vi "Untitled 7.vi"() -> ()   [LabVIEW 2019]
uses:
  <vilib>/Utility/file.llb/Read Delimited Spreadsheet (string).vi
panel:
  out "subarray 2":dbl[](array[numeric])=[0.124575, 0.249206, 0.374163, 0.498874, 0.623563, 0.748281, 0.872983, 0.997694, 1.12241, 1.247065, 1.371768, 1.496488, 1.621191, 1.745701, 1.870395, 1.995091, 2.119804, 2.244506, 2.369205]
  out "subarray":dbl[](array[numeric])=[204.971, 409.1489, 614.1025, 818.3818, 1022.829, 1226.951, 1431.292, 1635.939, 1840.247, 2044.703, 2248.928, 2453.218, 2657.61, 2861.815, 3066.024, 3270.177, 3474.445, 3679.15, 3883.288]
  out "appended array":string[][](array[string])=[["204.9710", "0.124575"], ["409.1489", "0.249206"], ["614.1025", "0.374163"], ["818.3818", "0.498874"], ["1022.829", "0.623563"], ["1226.951", "0.748281"], ["1431.292", "0.872983"], ["1635.939", "0.997694"], ["1840.247", "1.122410"], ["2044.703", "1.247065"], ["2248.928", "1.371768"], ["2453.218", "1.496488"], ["2657.610", "1.621191"], ["2861.815", "1.745701"], ["3066.024", "1.870395"], ["3270.177", "1.995091"], ["3474.445", "2.119804"], ["3679.150", "2.244506"], ["3883.288", "2.369205"]]
  out "all rows":string[][](array[string])
  in  "file path (dialog if empty)":path=path "D:/Projects/C2000/Grande/Data/ADC/Offset_Gain/Int_Ref_FCS_CHIP-2.txt"
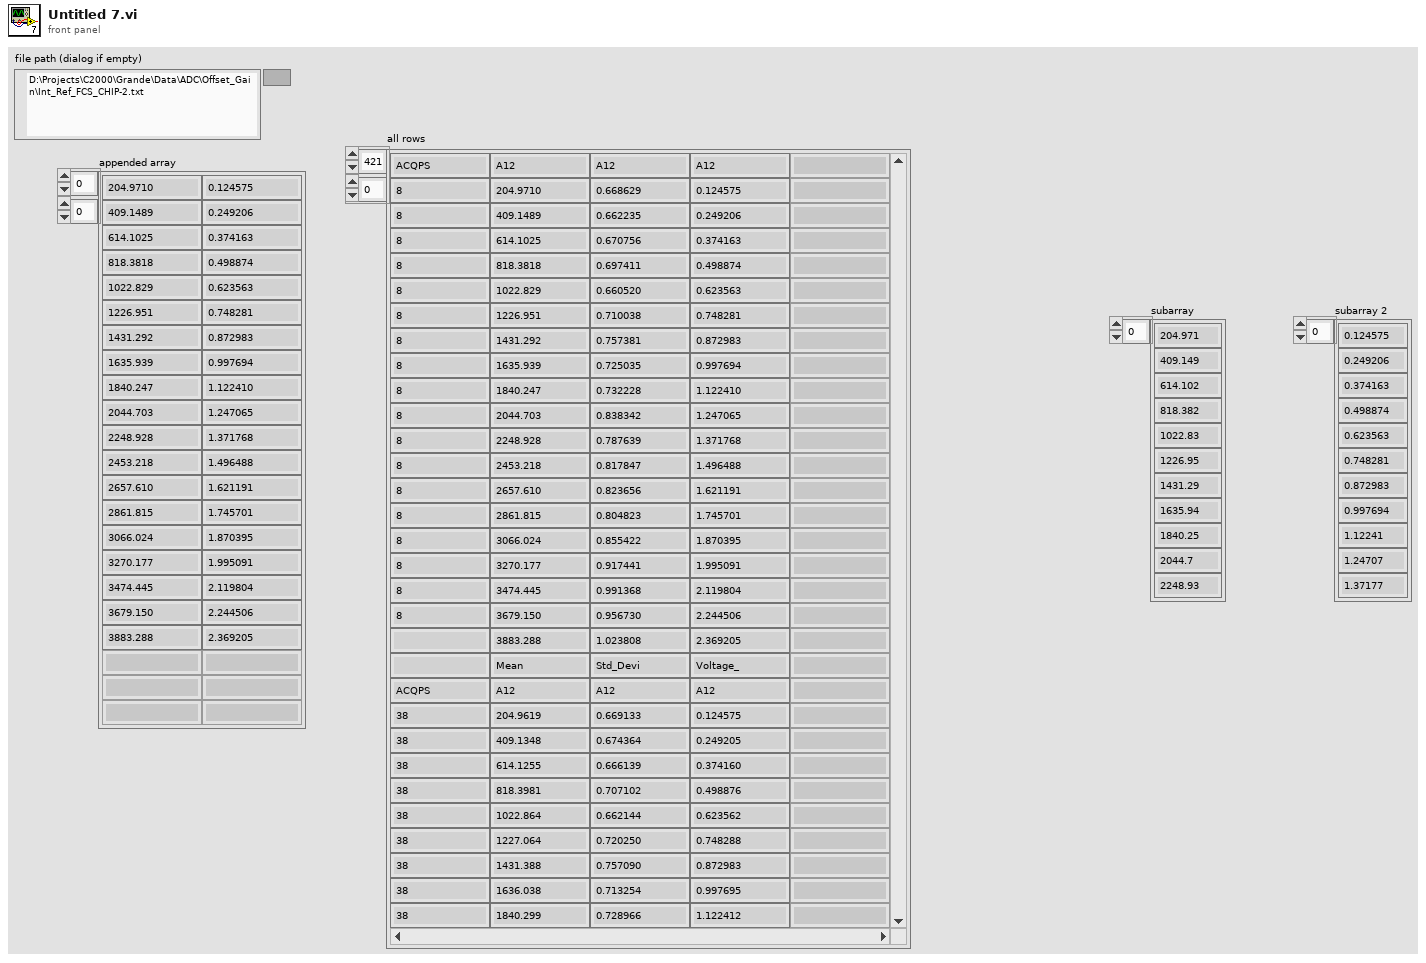
[diagram p1: front panel]
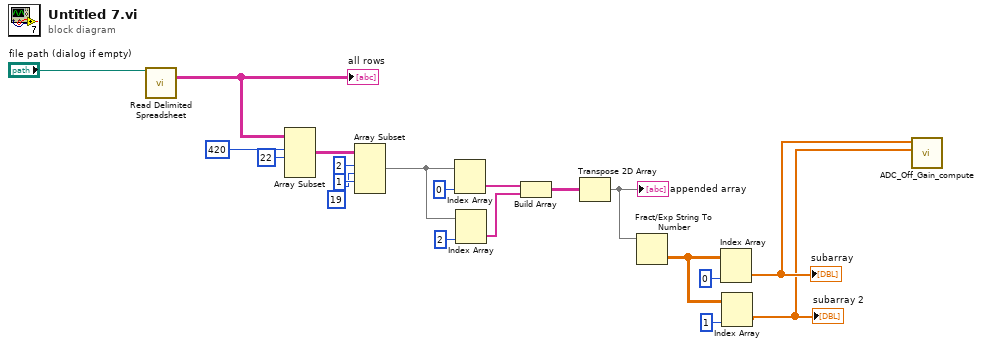
[diagram p0: block diagram]
diagram:
  n1 = call-poly <vilib>:"Read Delimited Spreadsheet.vi"("file path (dialog if empty)"="file path (dialog if empty)") -> ("all rows"=w19:string[][])  [unwired: 9 in, 5 out]
  "all rows" <- w19
  n2 = Array Subset(array=w19, index (row)=420 ("index"), length (row)=22 ("length")) -> (w15:string[][])  [unwired: 2 in]
  n3 = Array Subset(array=w15, index (row)=2 ("index"), length (row)=19 ("length"), index (col)=1 ("index")) -> (w12:string[][])  [unwired: 1 in]
  n4 = Index Array(array=w12, index (col)=0 ("disabled index (col)")) -> (element=w10:string[])  [unwired: 1 in]
  n5 = Index Array(array=w12, index (col)=2 ("disabled index (col)")) -> (element=w9:string[])  [unwired: 1 in]
  n6 = Build Array(w10, w9) -> (w8:string[][])
  n7 = Transpose 2D Array(2D array=w8) -> (transposed array=w6:string[][])
  "appended array" <- w6
  n8 = Fract/Exp String To Number(string=w6) -> (number=w5:dbl[][])  [unwired: 3 in, 1 out]
  n9 = Index Array(array=w5, index (col)=0 ("disabled index (col)")) -> (element=w2:dbl[])  [unwired: 1 in]
  "subarray" <- w2
  n10 = Index Array(array=w5, index (col)=1 ("disabled index (col)")) -> (element=w1:dbl[])  [unwired: 1 in]
  "subarray 2" <- w1
  n11 = call "ADC_Off_Gain_compute.vi"("Voltage_Array"=w1, "Code"=w2) -> ()  [unwired: 6 in, 4 out]
